vi "Main.vi"() -> ()   [LabVIEW 2020]
uses:
  <vilib>/Utility/config.llb/Read Key (Double).vi
  <vilib>/Utility/config.llb/NI_LVConfig.lvlib
panel:
  out "Run Time":dbl format="%<%M:%S>t"
  in  "Abort":bool
  out "LLB":path
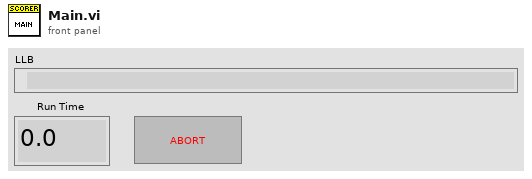
[diagram p1: front panel]
types:
  T1 = cluster{"Overall":dbl, "Categories":cluster{"Category":string, "Value":dbl}[]}
  T2 = typedef "NI_LVConfig.lvlib/Config Data RefNum.ctl" = refnum<k1>
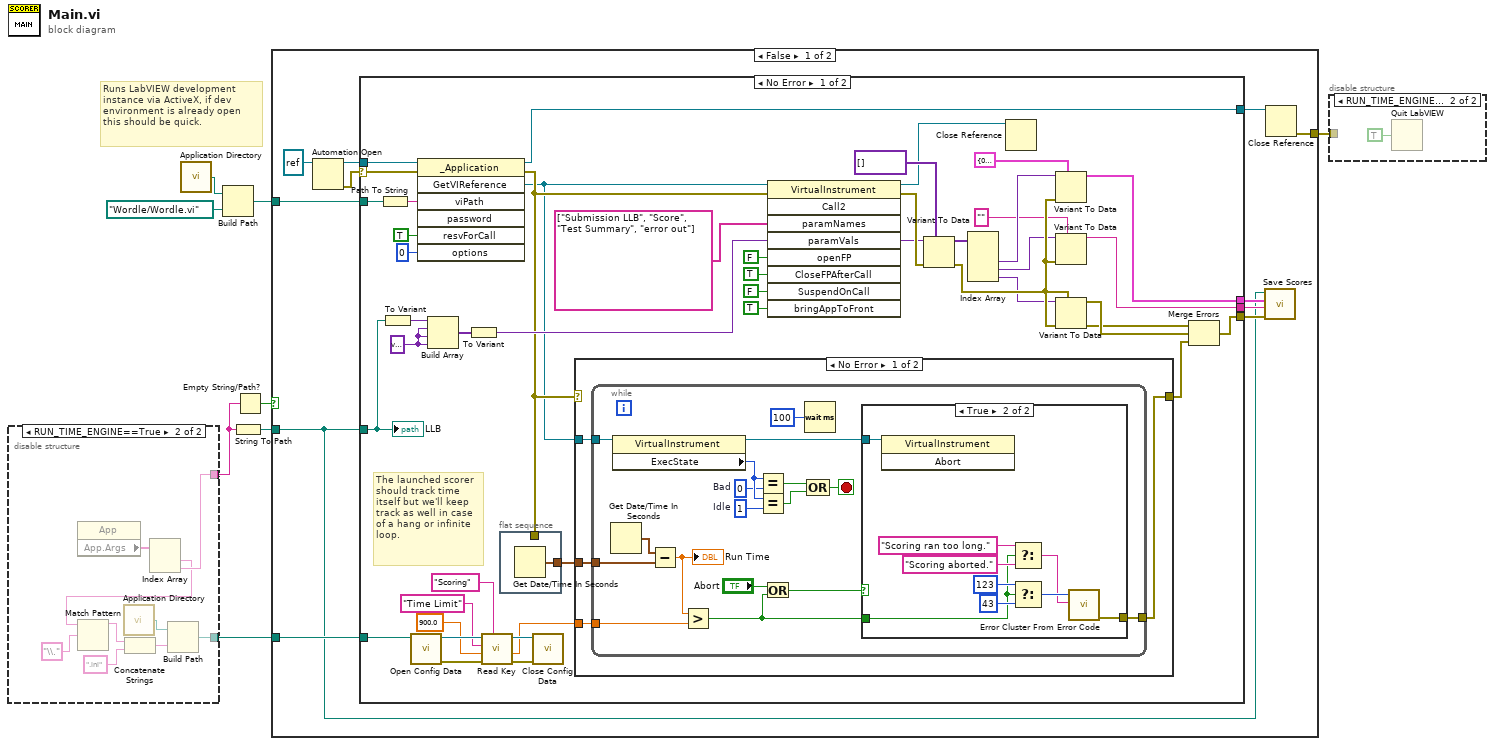
[diagram p0: block diagram]
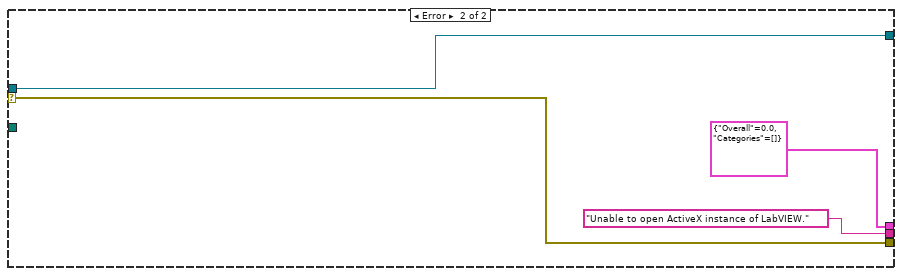
[diagram p4: hidden frame]
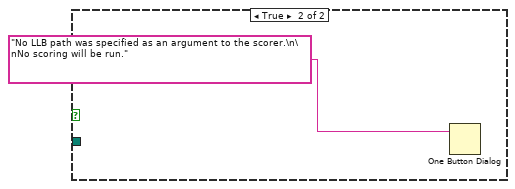
[diagram p5: hidden frame]
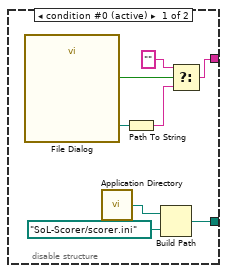
[diagram p6: hidden frame]
diagram:
  # "Runs LabVIEW development instance via ActiveX, if dev environment is already open this should be quick."
  n1 = disable-structure shown="RUN_TIME_ENGINE==True" {
    disable-tunnel: [w10 w24] -> w6
    disable-tunnel: [w15 w18] -> w5
    frame condition #0 (active) {
      n2 = call "File Dialog"() -> ("selected path"=w13:path, "cancelled"=w12:bool)  [unwired: 12 in, 2 out]
      n3 = call <vilib>:"Application Directory.vi"() -> ("Application Directory"=w16:path)
      n4 = Path To String(path=w13) -> (string=w11:string)
      n5 = Build Path(base path=w16, name or relative path=path "SoL-Scorer/scorer.ini") -> (appended path=w15:path)
      n6 = Select(t="", s=w12, f=w11) -> (s? t:f=w10:string)
    }
    frame condition #1 {
      n7 = property class="App"() -> ("App.Args"=w25:string[])  [unwired: 2 in, 2 out]
      n8 = call <vilib>:"Application Directory.vi"() -> ("Application Directory"=w22:path)
      n9 = Index Array(array=w25) -> (element #1=w17:string, element #2=w24:string)  [unwired: 2 in]
      n10 = Match Pattern(string=w17, regular expression="\\.") -> (before substring=w19:string)  [unwired: 1 in, 3 out]
      n11 = Concatenate Strings(w19, ".ini" ("string")) -> (w21:string)
      n12 = Build Path(base path=w22, name or relative path=w21) -> (appended path=w18:path)
    }
  }
  n13 = call <vilib>:"Application Directory.vi"() -> ("Application Directory"=w3:path)
  n14 = Build Path(base path=w3, name or relative path=path "Wordle/Wordle.vi") -> (appended path=w2:path)
  n15 = String To Path(string=w6) -> (path=w8:path)
  n16 = Empty String/Path?(string/path=w6) -> (empty?=w7:bool)
  n17 = case shown="False" w7 {
    tunnel: w2 -> [w35 _]
    tunnel: w8 -> [w26 _]
    tunnel: w5 -> [w32 _]
    tunnel: [w28 _] -> w4
    frame False {
      n18 = Automation Open(Automation Refnum=refnum<k7> refnum ("LabVIEW._Application")) -> (Automation Refnum=w27:refnum<k7>, error out=w36:errorcluster)  [unwired: 3 in]
      n19 = case shown="No Error" w36 {
        selector: w36 -> [w79 w115]
        tunnel: w35 -> [w64 _]
        tunnel: [w44 T1 {"Overall"=0.0, "Categories"=[]} ("Score")] -> w34
        tunnel: [w42 "Unable to open ActiveX instance of LabVIEW." ("Test Summary")] -> w33
        tunnel: w26 -> [w61 _]
        tunnel: w32 -> [w69 _]
        tunnel: [w68 w115] -> w31
        tunnel: w27 -> [w66 w118]
        tunnel: [w39 w118] -> w29
        frame No Error {
          w55 = variant
          # "The launched scorer should track time itself but we'll keep track as well in case of a hang or infinite loop."
          n20 = Path To String(path=w64) -> (string=w63:string)
          n21 = To Variant(anything=w61) -> (Variant=w56:variant)
          n22 = call <vilib>:"Open Config Data.vi"("configuration file path"=w69) -> ("error out"=w76:errorcluster, "refnum"=w77:T2)  [unwired: 8 in, 1 out]
          n23 = invoke class="_Application" method="GetVIReference"(reference=w66, error in=w79, "viPath"=w63, "resvForCall"=TRUE, "options"=0) -> (reference out=w39:refnum<k7>, error out=w38:errorcluster, "GetVIReference"=w37:refnum<k7>)  [unwired: 2 in, 4 out]
          n24 = Build Array(w56, w55, w55, w55) -> (w54:variant[])
          n25 = To Variant(anything=w54) -> (Variant=w52:variant)
          n26 = call-poly <vilib>:"Read Key.vi"("section"="Scoring", "error in (no error)"=w76, "default value"=900.0 ("y"), "key"="Time Limit" ("section"), "refnum"=w77) -> ("error out"=w71:errorcluster, "value"=w70:dbl, "refnum out"=w72:T2)  [unwired: 3 in, 1 out]
          n27 = flat-sequence {
            tunnel: [w83] -> w78
            tunnel: w38 -> [_]
            frame #0 {
              n28 = Get Date/Time In Seconds() -> (seconds since 1Jan1904=w83:timestamp)
            }
          }
          n29 = call <vilib>:"Close Config Data.vi"("error in (no error)"=w71, "refnum"=w72) -> ()  [unwired: 8 in, 2 out]
          n30 = case shown="No Error" w38 {
            selector: w38 -> [_ w114]
            tunnel: w78 -> [w87 _]
            tunnel: w70 -> [w86 _]
            tunnel: [w84 w114] -> w67
            tunnel: w37 -> [w85 _]
            frame No Error {
              n31 = while {
                tunnel: w87 -> [w103]
                tunnel: w86 -> [w100]
                tunnel: w85 -> [w89]
                tunnel: [w88] -> w84
                stop <- w98 stop-if-true
                w90 = 1  # Idle
                w91 = 0  # Bad
                n32 = Get Date/Time In Seconds() -> (seconds since 1Jan1904=w102:timestamp)
                n33 = property class="VirtualInstrument"(reference=w89) -> (reference out=w97:refnum<k7>, "ExecState"=w93:i32)  [unwired: 1 in, 1 out]
                n34 = Subtract(x=w102, y=w103) -> (x-y=w101:dbl)
                "Run Time" <- w101
                n35 = Greater?(x=w101, y=w100) -> (0:w94:bool)
                n36 = Equal?(x=w93, y=w91) -> (x = y?=w99:bool)
                n37 = Equal?(x=w93, y=w90) -> (x = y?=w92:bool)
                n38 = Or(x="Abort", y=w94) -> (x .or. y?=w95:bool)
                n39 = Wait (ms)(milliseconds to wait=u32 100) -> ()  [unwired: 1 out]
                n40 = Compound Arithmetic op=OR(w99, w92) -> (w98:bool)
                n41 = case shown="True" w95 {
                  tunnel: w97 -> [_ w106]
                  tunnel: w94 -> [_ w108]
                  tunnel: [_ w105] -> w88
                  frame False {
                  }
                  frame True {
                    n42 = invoke class="VirtualInstrument" method="Abort"(reference=w106) -> ()  [unwired: 2 in, 3 out]
                    n43 = Select(t="Scoring ran too long." ("error message (\"\")"), s=w108, f="Scoring aborted." ("error message (\"\")")) -> (s? t:f=w107:string)
                    n44 = Select(t=123 ("error code (0)"), s=w108, f=43 ("error code (0)")) -> (s? t:f=w111:i32)
                    n45 = call <vilib>:"Error Cluster From Error Code.vi"("error message (\"\")"=w107, "error code (0)"=w111) -> ("error out"=w105:errorcluster)  [unwired: 7 in]
                  }
                }
              }
            }
            frame Error {
            }
          }
          n46 = invoke class="VirtualInstrument" method="Call2"(reference=w37, error in=w38, "paramNames"=string[] ["Submission LLB", "Score", "Test Summary", "error out"], "paramVals"=w52, "openFP"=FALSE, "CloseFPAfterCall"=TRUE, "SuspendOnCall"=FALSE, "bringAppToFront"=TRUE) -> (reference out=w40:refnum<k7>, error out=w82:errorcluster, "paramVals"=w51:variant)  [unwired: 1 in, 6 out]
          n47 = Variant To Data(error in=w82, type=variant[] [], Variant=w51) -> (data=w49:variant[], error out=w80:errorcluster)
          n48 = Index Array(array=w49) -> (element #2=w46:variant, element #3=w47:variant, element #4=w48:variant)  [unwired: 4 in, 1 out]
          n49 = Close Reference(reference=w40) -> ()  [unwired: 1 in, 1 out]
          n50 = Variant To Data(error in=w80, type=T1 {"Overall"=0.0, "Categories"=[]} ("Score"), Variant=w46) -> (data=w44:T1)  [unwired: 1 out]
          n51 = Variant To Data(error in=w80, type="", Variant=w47) -> (data=w42:string)  [unwired: 1 out]
          n52 = Variant To Data(error in=w80, type=w80, Variant=w48) -> (data=w81:errorcluster, error out=w41:errorcluster)
          n53 = Merge Errors(w41, w81, w67) -> (w68:errorcluster)
          "LLB" <- w61
        }
        frame Error {
        }
      }
      n54 = call "Save Scores.vi"("error in (no error)"=w31, "Test Summary"=w33, "Score"=w34, "LLB Path"=w26) -> ()  [unwired: 7 in, 1 out]
      n55 = Close Reference(reference=w29) -> (error out=w28:errorcluster)  [unwired: 1 in]
    }
    frame True {
      n56 = One Button Dialog(message="No LLB path was specified as an argument to the scorer.\n\nNo scoring will be run.") -> ()  [unwired: 1 in, 1 out]
    }
  }
  n57 = disable-structure shown="RUN_TIME_ENGINE==True" {
    disable-tunnel: w4 -> [_ _]
    frame condition #0 (active) {
    }
    frame condition #1 {
      n58 = Quit LabVIEW(quit? (T)=TRUE) -> ()
    }
  }
